vi "MainVI.vi"() -> ()   [LabVIEW 2021]
uses:
  <vilib>/MakerHub/LINX/Public/Peripherals/Digital/Digital Write 1 Chan.vi
  <vilib>/MakerHub/LINX/Public/Peripherals/Digital/Digital Write N Chans.vi
  <vilib>/MakerHub/LINX/Private/Local IO/LinxDigitalWrite.vi
  <vilib>/MakerHub/LINX/Public/Utilities/Check Channel.vi
  <vilib>/MakerHub/LINX/Private/Local IO/Handle Errors.vi
  <vilib>/MakerHub/LINX/Public/Utilities/Open Local.vi
  <vilib>/MakerHub/LINX/Private/Utilties/Generate Error.vi
  <vilib>/MakerHub/LINX/LMH-LINX.lvlib
  <vilib>/ptbypt/NI_PtbyPt.lvlib
panel:
  out "Array":bool[](array[boolean])
  in  "stop":bool
  out "Temperatura ºC":dbl
  out "Temperatura Real":dbl(graph)
  out "Device Name":string
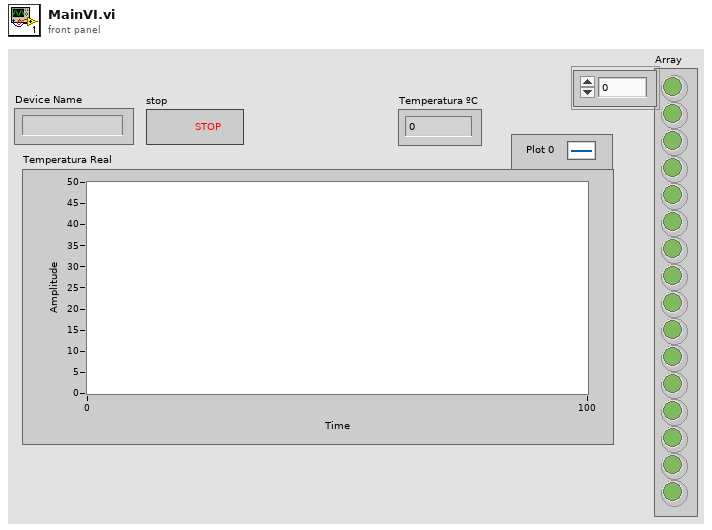
[diagram p1: front panel]
types:
  T1 = typedef "LMH-LINX.lvlib/LINX Ref.ctl" = cluster{"IO":T2, "Interface":T3, "LINX Device Config":T4}
  T2 = typedef "LMH-LINX.lvlib/Platform.ctl" = enum16{"Remote", "Local"}
  T3 = typedef "LMH-LINX.lvlib/Interface.ctl" = enum16{"Serial", "TCP"}
  T4 = typedef "LMH-LINX.lvlib/Device.lvlib/LINX Device Config.ctl" = cluster{"Interface":T3, "COM Port":refnum<visa-resource-name>, "TCP Configuration":T5, "Device Family":u8, "Device ID":u8, "Device Name":string, "TCP Ref":refnum<k5>, "Channels":T6}
  T5 = typedef "LMH-LINX.lvlib/Device.lvlib/TCP Config.ctl" = cluster{"IP Address":string, "Port":u16}
  T6 = typedef "LMH-LINX.lvlib/Channels.ctl" = cluster{"DI":u8[], "DO":u8[], "AI":u8[], "AO":u8[], "PWM":u8[], "QE":u8[], "UART":u8[], "I2C 2":u8[], "SPI":u8[], "CAN":u8[], "Servo":u8[], "AI Ref (V)":dbl, "AI Resolution (Bits)":u8, "AO Ref (V)":dbl, "AO Resolution (Bits)":u8}
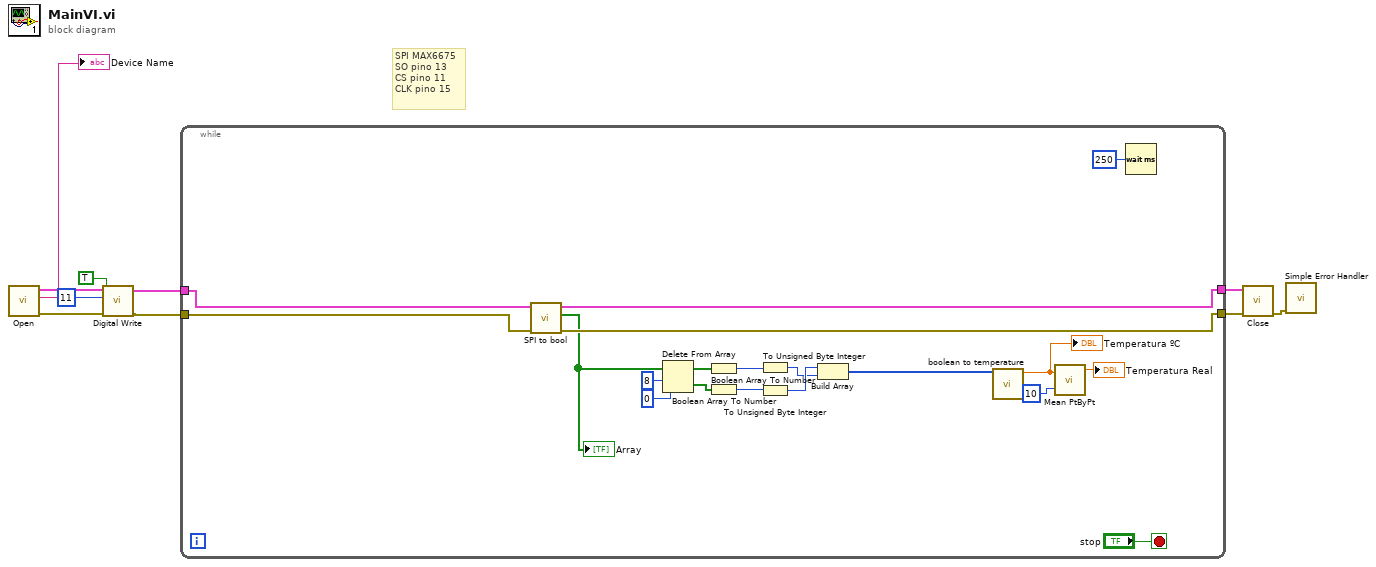
[diagram p0: block diagram]
diagram:
  # "SPI MAX6675\nSO pino 13\nCS pino 11\nCLK pino 15"
  n1 = call-poly <vilib>:"Open.vi"() -> ("Error Out"=w7:errorcluster, "Device Name"=→"Device Name":string, "LINX Resource"=w8:T1)  [unwired: 9 in]
  n2 = call-poly <vilib>:"Digital Write.vi"("Error In"=w7, "Output Value"=TRUE, "DO Channel"=u8 11, "LINX Resource"=w8) -> ("Error Out"=w3:errorcluster, "LINX Resource"=w4:T1)  [unwired: 6 in]
  n3 = while {
    tunnel: w4 -> [w24]
    tunnel: w3 -> [w23]
    tunnel: [w22] -> w2
    tunnel: [w21] -> w1
    stop <- "stop" stop-if-true
    n4 = call "SPI to bool.vi"("error in (no error)"=w23, "LINX Resource in"=w24) -> ("error out"=w21:errorcluster, "Array"=w20:bool[], "LINX Resource out"=w22:T1)  [unwired: 7 in]
    "Array" <- w20
    n5 = Delete From Array(array=w20, length=8, index=0) -> (deleted portion=w16:bool[], array with subset deleted=w17:bool[])
    n6 = Boolean Array To Number(Boolean array=w17) -> (number=w15:u32)
    n7 = Boolean Array To Number(Boolean array=w16) -> (number=w14:u32)
    n8 = To Unsigned Byte Integer(number=w15) -> (unsigned 8bit integer=w11:u8)
    n9 = To Unsigned Byte Integer(number=w14) -> (unsigned 8bit integer=w12:u8)
    n10 = Build Array(w12, w11) -> (w13:u8[])
    n11 = call "boolean to temperature.vi"("SPI array"=w13) -> ("Temperatura"=w27:dbl)  [unwired: 10 in]
    "Temperatura ºC" <- w27
    n12 = call <vilib>:"Mean PtByPt.vi"("x"=w27, "sample length"=10) -> ("mean"=→"Temperatura Real":dbl)  [unwired: 2 in, 1 out]
    n13 = Wait (ms)(milliseconds to wait=u32 250) -> ()  [unwired: 1 out]
  }
  n14 = call <vilib>:"Close.vi"("Error In"=w1, "LINX Resource"=w2) -> ("Error Out"=w9:errorcluster)  [unwired: 9 in]
  n15 = call <vilib>:"Simple Error Handler.vi"("error in (no error)"=w9) -> ()  [unwired: 4 in, 5 out]
